vi "Flex Editor Context.vi"() -> (2 "Flex Editor Context":string="ig.flex.editor")   [LabVIEW 2022 SP3, in "FlexBlocks Support.lvlib"]
uses:
  FlexBlocks Support.lvlib
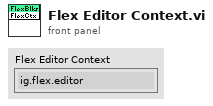
[diagram p1: front panel]
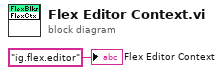
[diagram p0: block diagram]
diagram:
  "Flex Editor Context" <- "ig.flex.editor" ("Application Instance Name")
